vi "Set Font.vi"(7 "Sheet Name":string, 8 "error in":errorcluster, 9 "Font":T1={"Bold"=enum."default", "Italic"=enum."default", "Underline"=enum."default", "TextColor"=0, "TextSize"=-1.0, "Name"=""}, 10 "Cell Address":string, 11 "SpreadsheetDoc in":refnum<k24>) -> (0 "error out":errorcluster, 3 "SpreadsheetDoc out":refnum<k24>)   [LabVIEW 2019, in "Open Xml.lvlib"]
uses:
  Open Xml.lvlib
  D:/git/Open-Xml-LabVIEW/Source/DocumentFormat.OpenXml.dll
  DocumentFormat.OpenXml.dll
  Font.ctl
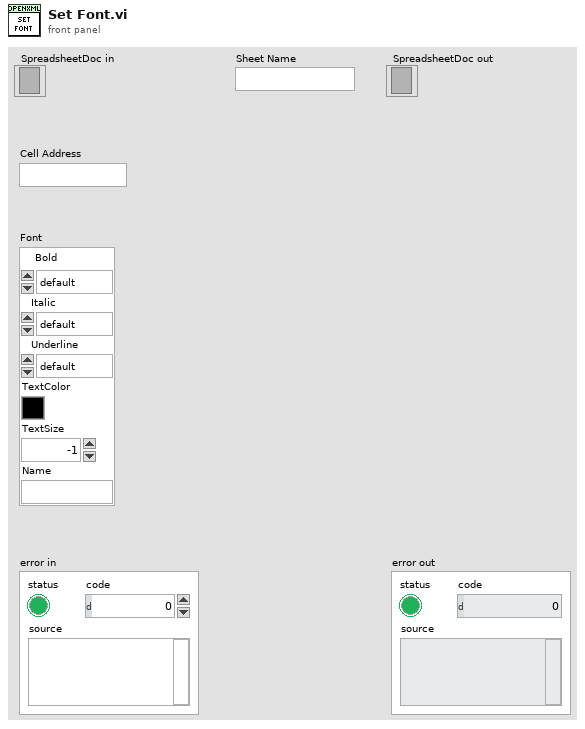
[diagram p1: front panel]
types:
  T1 = typedef "Open Xml.lvlib/Font.ctl" = cluster{"Bold":enum16{"bold", "regular", "default"}, "Italic":enum16{"italic", "regular", "default"}, "Underline":enum16{"single", "double", "singleAccounting", "doubleAccounting", "none", "default"}, "TextColor":u32, "TextSize":dbl, "Name":string}
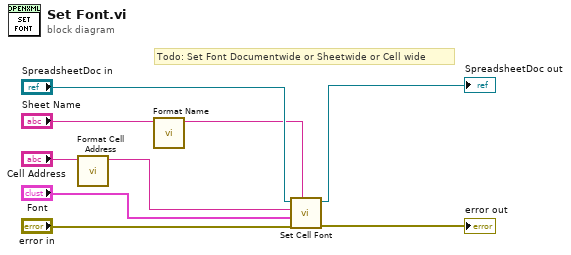
[diagram p0: block diagram]
diagram:
  # "Todo: Set Font Documentwide or Sheetwide or Cell wide"
  n1 = call "Format Cell Address.vi"("Cell Address"="Cell Address") -> ("Formatted Cell Address"=w1:string)  [unwired: 10 in]
  n2 = call "Format Name.vi"("Sheet Name"="Sheet Name") -> ("Formatted Sheet Name"=w2:string)  [unwired: 10 in]
  n3 = call "Set Cell Font.vi"("Sheet Name"=w2, "error in"="error in", "Font"="Font", "Cell Address"=w1, "SpreadsheetDoc in"="SpreadsheetDoc in") -> ("error out"=→"error out":errorcluster, "SpreadsheetDoc out"=→"SpreadsheetDoc out":refnum<k24>)  [unwired: 5 in]
